vi "container.vi"() -> ()   [LabVIEW 2009]
panel:
  out "string":string
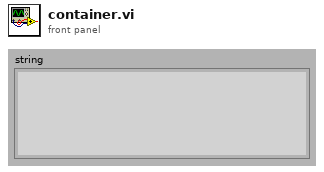
[diagram p1: front panel]
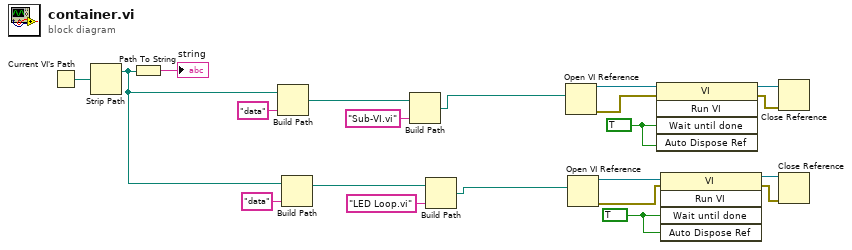
[diagram p0: block diagram]
diagram:
  w8 = TRUE ("Wait Until Done")
  w11 = TRUE ("Wait Until Done")
  n1 = Current VI's Path() -> (path=w20:path)
  n2 = Strip Path(path=w20) -> (stripped path=w17:path)  [unwired: 1 out]
  n3 = Path To String(path=w17) -> (string=→"string":string)
  n4 = Build Path(base path=w17, name or relative path="data") -> (appended path=w15:path)
  n5 = Build Path(base path=w17, name or relative path="data") -> (appended path=w2:path)
  n6 = Build Path(base path=w15, name or relative path="Sub-VI.vi") -> (appended path=w14:path)
  n7 = Build Path(base path=w2, name or relative path="LED Loop.vi") -> (appended path=w1:path)
  n8 = Open VI Reference(vi path=w14) -> (vi reference=w12:refnum<vi>, error out=w13:errorcluster)  [unwired: 5 in]
  n9 = Open VI Reference(vi path=w1) -> (vi reference=w10:refnum<vi>, error out=w9:errorcluster)  [unwired: 5 in]
  n10 = invoke class="VI" method="Run VI"(reference=w12, error in=w13, "Wait until done"=w11, "Auto Dispose Ref"=w11) -> (reference out=w6:refnum<vi>, error out=w7:errorcluster)  [unwired: 1 in, 3 out]
  n11 = invoke class="VI" method="Run VI"(reference=w10, error in=w9, "Wait until done"=w8, "Auto Dispose Ref"=w8) -> (reference out=w4:refnum<vi>, error out=w5:errorcluster)  [unwired: 1 in, 3 out]
  n12 = Close Reference(reference=w6, error in (no error)=w7) -> ()  [unwired: 1 out]
  n13 = Close Reference(reference=w4, error in (no error)=w5) -> ()  [unwired: 1 out]
